vi "Get passive targets.vi"(11 "PN532 COM Port":refnum<visa-resource-name>) -> (0 "error out":errorcluster, 1 "NFC ID (ASCII)":string, 2 "Found?":bool, 3 "PN532 COM Port Out":refnum<visa-resource-name>, 5 "NFC ID (HEX)":string)   [LabVIEW 2012, in "NFC Driver.lvlib"]
uses:
  NFC Driver.lvlib
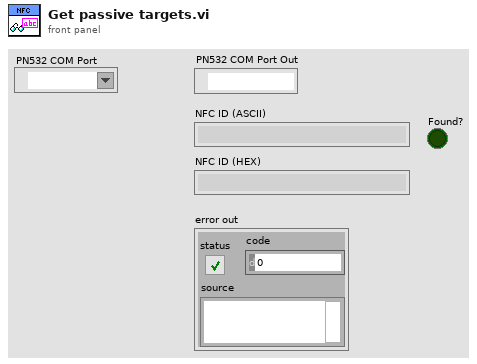
[diagram p1: front panel]
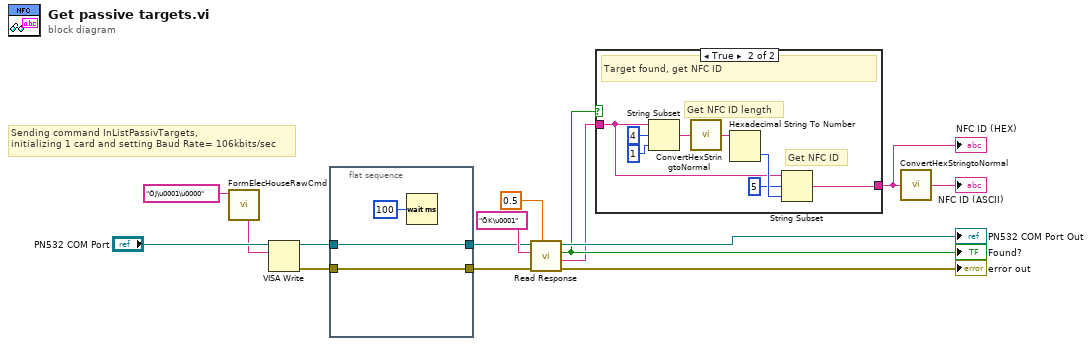
[diagram p0: block diagram]
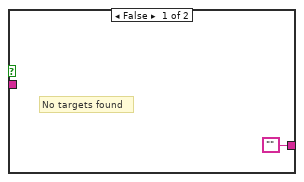
[diagram p2: hidden frame]
diagram:
  # "Sending command InListPassivTargets,\ninitializing 1 card and setting Baud Rate= 106kbits/sec"
  n1 = call "FormElecHouseRawCmd.vi"("Command"="ÔJ\u0001\u0000") -> ("concatenated Cmd"=w13:string)  [unwired: 10 in]
  n2 = VISA Write(VISA resource name="PN532 COM Port", write buffer=w13) -> (VISA resource name out=w4:refnum<visa-resource-name>, error out=w2:errorcluster)  [unwired: 1 in, 1 out]
  n3 = flat-sequence {
    tunnel: w4 -> [w17]
    tunnel: [w17] -> w3
    tunnel: w2 -> [w16]
    tunnel: [w16] -> w1
    frame #0 {
      n4 = Wait (ms)(milliseconds to wait=u32 100) -> ()  [unwired: 1 out]
    }
  }
  n5 = call "Read Response.vi"("Timeout (s)"=0.5, "error in (no error)"=w1, "regular expression"="ÕK\u0001", "PN532 COM Port"=w3) -> ("error out"=→"error out":errorcluster, "Response Data"=w8:string, "Found?"=w9:bool, "PN532 COM Port Out"=→"PN532 COM Port Out":refnum<visa-resource-name>)  [unwired: 4 in]
  "Found?" <- w9
  n6 = case shown="True" w9 {
    tunnel: w8 -> [_ w21]
    tunnel: ["" w20] -> w5
    frame False {
      # "No targets found"
    }
    frame True {
      # "Get NFC ID"
      # "Get NFC ID length"
      # "Target found, get NFC ID"
      n7 = String Subset(string=w21, offset (0)=4, length (rest)=1 ("length (rest)")) -> (substring=w26:string)
      n8 = call "ConvertHexStringtoNormal.vi"("Hex String"=w26) -> ("Normal String"=w25:string)
      n9 = Hexadecimal String To Number(string=w25) -> (number=w23:u32)  [unwired: 2 in, 1 out]
      n10 = String Subset(string=w21, offset (0)=5, length (rest)=w23) -> (substring=w20:string)
    }
  }
  "NFC ID (HEX)" <- w5
  n11 = call "ConvertHexStringtoNormal.vi"("Hex String"=w5) -> ("Normal String"=→"NFC ID (ASCII)":string)
